vi "init.vi"(8 "error in (no error)":errorcluster, 11 "Glaz-I in":refnum<class "Glaz.lvclass">) -> (0 "error out":errorcluster, 3 "Glaz-I out":refnum<class "Glaz.lvclass">)   [LabVIEW 2019, in "Glaz.lvclass"]
uses:
  Glaz.lvclass
  _cameraBase/_cameraBase.lvclass
  <userlib>/GlazLabView/GlazLib.lvlib
panel:
  out "Hardware Version":string
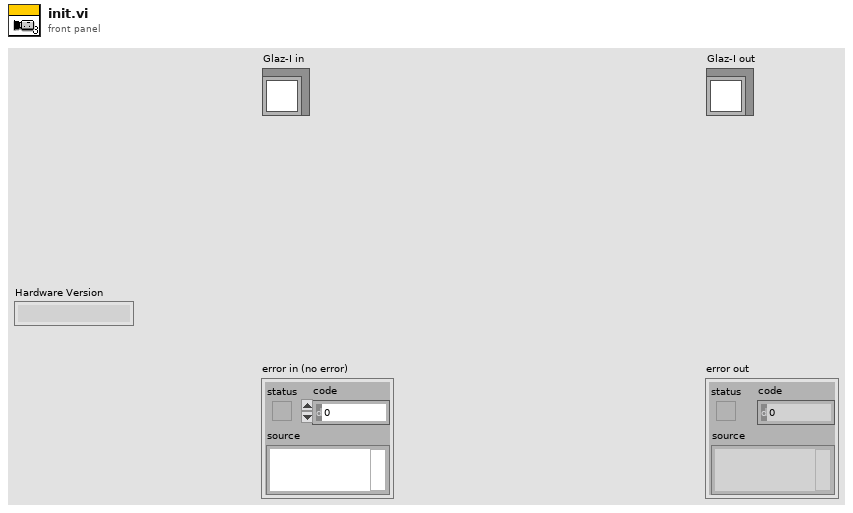
[diagram p1: front panel]
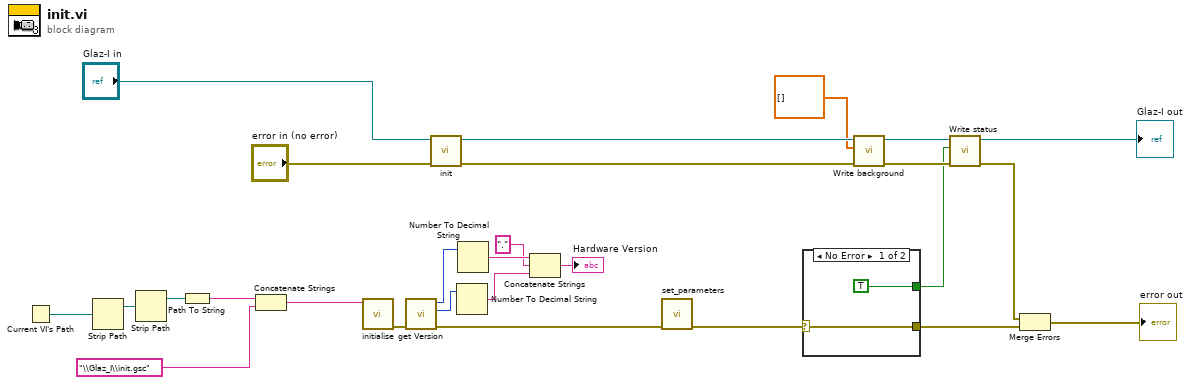
[diagram p0: block diagram]
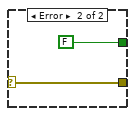
[diagram p2: hidden frame]
diagram:
  n1 = Current VI's Path() -> (path=w6:path)
  n2 = Strip Path(path=w6) -> (stripped path=w5:path)  [unwired: 1 out]
  n3 = Strip Path(path=w5) -> (stripped path=w4:path)  [unwired: 1 out]
  n4 = Path To String(path=w4) -> (string=w3:string)
  n5 = Concatenate Strings(w3, "\\Glaz_I\\init.gsc") -> (w1:string)
  n6 = call <userlib>:"initialise.vi"("scriptFileName"=w1) -> ("error out"=w21:errorcluster)  [unwired: 9 in, 1 out]
  n7 = call <userlib>:"get Version.vi"("error in (no error)"=w21) -> ("error out"=w19:errorcluster, "minorVersion"=w23:i32, "majorVersion"=w22:i32)  [unwired: 8 in]
  n8 = call-parent "init.vi"("error in (no error)"="error in (no error)", "_cameraBase in"="Glaz-I in") -> ("error out"=w15:errorcluster, "_cameraBase out"=w17:refnum<class "Glaz.lvclass">)  [unwired: 8 in]
  n9 = Number To Decimal String(number=w23) -> (decimal integer string=w26:string)  [unwired: 1 in]
  n10 = Number To Decimal String(number=w22) -> (decimal integer string=w24:string)  [unwired: 1 in]
  n11 = Concatenate Strings(w24, "." ("string"), w26) -> (→"Hardware Version":string)
  n12 = call "set_parameters.vi"("error in (no error)"=w19) -> ("error out (no error)"=w13:errorcluster)  [unwired: 10 in]
  n13 = case shown="No Error" w13 {
    selector: w13 -> [w29 w31]
    tunnel: [w29 w31] -> w12
    tunnel: [TRUE FALSE] -> w7
    frame No Error {
    }
    frame Error {
    }
  }
  n14 = call-dynamic "Write background.vi"("error in (no error)"=w15, "background"=dbl[] [], "Glaz-I in"=w17) -> ("error out"=w10:errorcluster, "Glaz-I out"=w11:refnum<class "Glaz.lvclass">)  [unwired: 7 in]
  n15 = call-dynamic "Write status.vi"("error in (no error)"=w10, "status"=w7, "_cameraBase in"=w11) -> ("error out"=w8:errorcluster, "_cameraBase out"=→"Glaz-I out":refnum<class "Glaz.lvclass">)  [unwired: 7 in]
  n16 = Merge Errors(w8, w12) -> (→"error out":errorcluster)
